vi "点到直线距离.vi"(10 "Straight Edge (X)":T1, 11 "簇":cluster{"Numeric":dbl, "Numeric":dbl}) -> (1 "Distance":dbl format="%.2f", 2 "垂点":cluster{"X":sgl, "Y":sgl}, 3 "Perpendicular Line":T2)   [LabVIEW 2014]
uses:
  <vilib>/vision/NI_Vision_Development_Module.lvlib
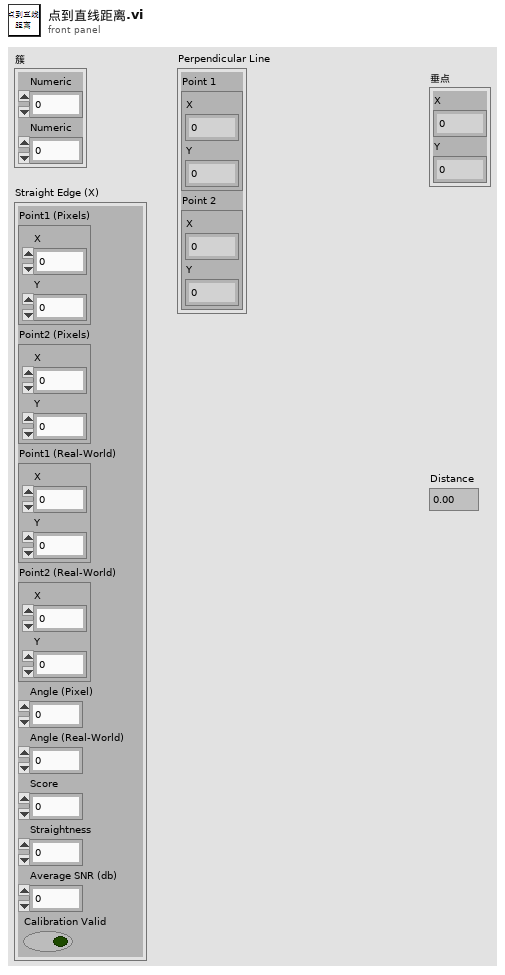
[diagram p1: front panel]
types:
  T1 = cluster{"Point1 (Pixels)":cluster{"X":sgl, "Y":sgl}, "Point2 (Pixels)":cluster{"X":sgl, "Y":sgl}, "Point1 (Real-World)":cluster{"X":sgl, "Y":sgl}, "Point2 (Real-World)":cluster{"X":sgl, "Y":sgl}, "Angle (Pixel)":dbl, "Angle (Real-World)":dbl, "Score":dbl, "Straightness":dbl, "Average SNR (db)":dbl, "Calibration Valid":bool}
  T2 = cluster{"Point 1":cluster{"X":sgl, "Y":sgl}, "Point 2":cluster{"X":sgl, "Y":sgl}}
  T3 = cluster{"Point1 (Pixels)":cluster{"X":sgl, "Y":sgl}, "Point2 (Pixels)":cluster{"X":sgl, "Y":sgl}}
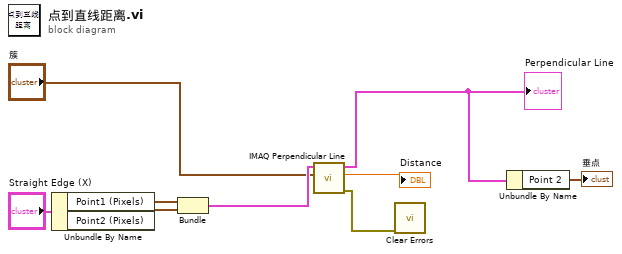
[diagram p0: block diagram]
diagram:
  n1 = Unbundle By Name("Straight Edge (X)") -> ("Point1 (Pixels)"=w7:cluster{"X":sgl, "Y":sgl}, "Point2 (Pixels)"=w6:cluster{"X":sgl, "Y":sgl})
  n2 = Bundle("Point1 (Pixels)"=w7, "Point2 (Pixels)"=w6) -> (w8:T3)  [unwired: 1 in]
  n3 = call "IMAQ Perpendicular Line"("Point"="簇", "Line"=w8) -> ("error out"=w1:errorcluster, "Distance"=→"Distance":dbl, "Perpendicular Line"=w3:T2)  [unwired: 7 in]
  "Perpendicular Line" <- w3
  n4 = call <vilib>:"Clear Errors.vi"("error in (no error)"=w1) -> ()  [unwired: 5 in, 2 out]
  n5 = Unbundle By Name(w3) -> ("Point 2"=→"垂点":cluster{"X":sgl, "Y":sgl})
